vi "Update Relays.vi"(8 "error in (no error)":errorcluster, 10 "MUX Section Ref in":T1 format="%.0x", 11 "Selected MUX Relays":refnum<vi>) -> (0 "error out":errorcluster)   [LabVIEW 2013, in "MUX Custom Device.lvlib"]
uses:
  MUX Custom Device.lvlib
  <vilib>/NI Veristand/Custom Device API/Custom Device Item Ref.ctl
  Relay Channel Data.ctl
  Relay Data.ctl
  Switch.ctl
  MUX Global.vi
  <vilib>/NI Veristand/Custom Device API/Get Item Property (String).vi
  <vilib>/NI Veristand/Custom Device Tools/Custom Device Utility Library/Custom Device Utility Library.lvlib
  <vilib>/NI Veristand/Custom Device API/Custom Device API.lvlib
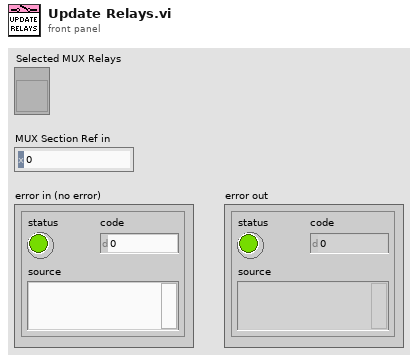
[diagram p1: front panel]
types:
  T1 = typedef "Custom Device API.lvlib/Custom Device Item Ref.ctl" = u64
  T2 = typedef "Relay Status.ctl" = cluster{"Present":bool, "Relay Data":T3}
  T3 = typedef "MUX Custom Device.lvlib/Relay Data.ctl" = cluster{"Relay Name":string, "State":T4}
  T4 = typedef "MUX Custom Device.lvlib/Switch.ctl" = bool
  T5 = typedef "MUX Custom Device.lvlib/Relay Status.ctl" = cluster{"Present":bool, "Relay Data":T3}
  T6 = typedef "MUX Custom Device.lvlib/Relay Channel Data.ctl" = cluster{"Relay Channel Name":string, "Relay Data":T3}
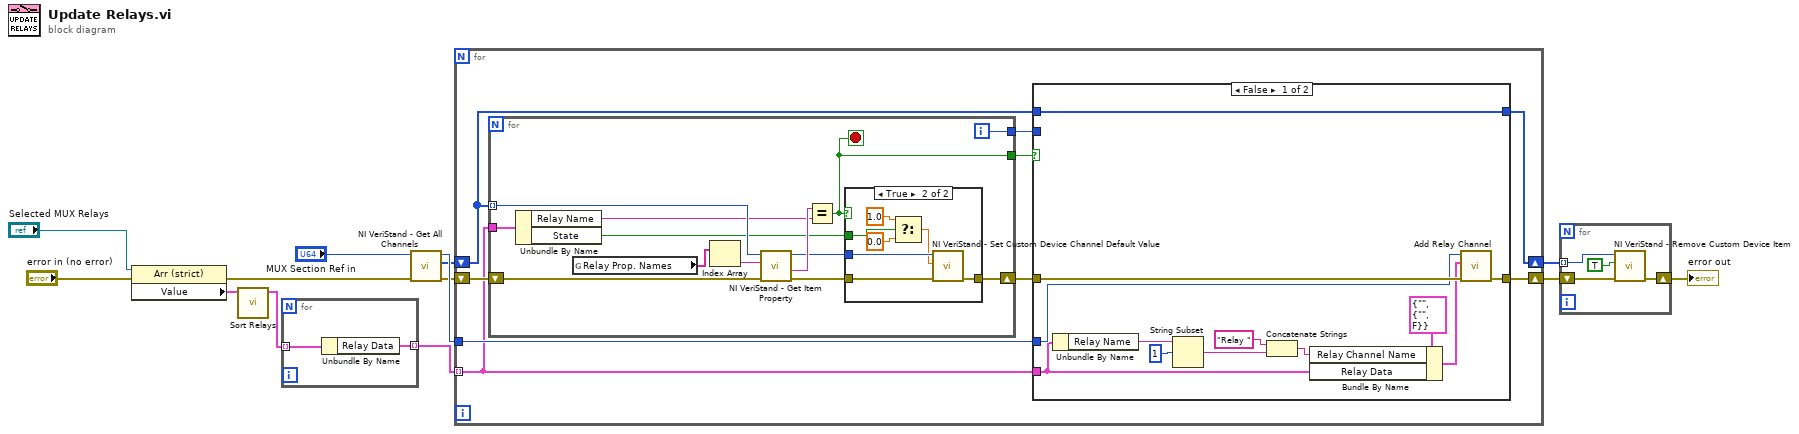
[diagram p0: block diagram]
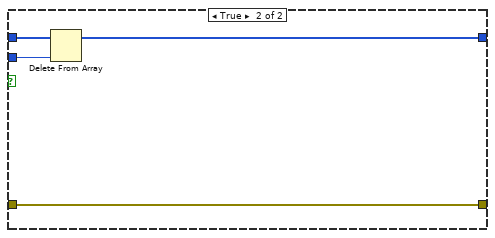
[diagram p2: hidden frame]
diagram:
  n1 = property class="Arr (strict)"(reference="Selected MUX Relays", error in="error in (no error)") -> (error out=w1:errorcluster, "Value"=w12:T2[])  [unwired: 1 out]
  n2 = call "Sort Relays.vi"("Relays"=w12) -> ("Sorted Relays"=w13:T5[])  [unwired: 10 in]
  n3 = for {
    tunnel: w13 -> [w15] mode=indexing
    tunnel: [w14] -> w7 mode=indexing
    n4 = Unbundle By Name(w15) -> ("Relay Data"=w14:T3)
  }
  n5 = call <vilib>:"NI VeriStand - Get All Channels.vi"("error in"=w1, "Section Ref in"="MUX Section Ref in") -> ("error out"=w6:errorcluster, "Channel Refs"=w5:T1[], "Section Ref out"=w8:T1)  [unwired: 6 in, 1 out]
  n6 = for {
    shift-right: [w22] -> w10
    shift-left: w5 -> [w23]
    tunnel: w7 -> [w18] mode=indexing
    tunnel: w8 -> [w20]
    shift-right: [w19] -> w9
    shift-left: w6 -> [w24]
    n7 = for {
      tunnel: w23 -> [w53] mode=indexing
      tunnel: w18 -> [w48]
      shift-right: [w44] -> w21
      shift-left: w24 -> [w49]
      tunnel: [w42] -> w17
      tunnel: [w41] -> w16
      i -> [w42]
      stop <- w41 stop-if-true
      n8 = Unbundle By Name(w48) -> ("Relay Name"=w47:string, "State"=w43:T4)
      n9 = global read "MUX Global.vi" "Relay Prop. Names"() -> (w52:string[])
      n10 = Index Array(array=w52) -> (element=w51:string)  [unwired: 1 in]
      n11 = call-poly <vilib>:"NI VeriStand - Get Item Property.vi"("error in (no error)"=w49, "Property Name"=w51, "Item Ref in"=w53) -> ("error out"=w46:errorcluster, "Value"=w50:string, "Item Ref out"=w45:T1)  [unwired: 5 in, 1 out]
      n12 = Equal?(x=w50, y=w47) -> (x = y?=w41:bool)
      n13 = case shown="True" w41 {
        tunnel: w46 -> [w54 w61]
        tunnel: w45 -> [_ w60]
        tunnel: [w54 w59] -> w44
        tunnel: w43 -> [_ w58]
        frame False {
        }
        frame True {
          n14 = Select(t=1.0, s=w58, f=0.0) -> (s? t:f=w55:dbl)
          n15 = call <vilib>:"NI VeriStand - Set Custom Device Channel Default Value.vi"("error in (no error)"=w61, "Default Value"=w55, "Channel Ref in"=w60) -> ("error out"=w59:errorcluster)  [unwired: 7 in, 1 out]
        }
      }
    }
    n16 = case shown="False" w16 {
      tunnel: w23 -> [w36 w40]
      tunnel: [w36 w39] -> w22
      tunnel: w21 -> [w35 w37]
      tunnel: w20 -> [w34 _]
      tunnel: [w33 w37] -> w19
      tunnel: w18 -> [w30 _]
      tunnel: w17 -> [_ w38]
      frame False {
        n17 = Unbundle By Name(w30) -> ("Relay Name"=w29:string)
        n18 = String Subset(string=w29, offset (0)=1) -> (substring=w27:string)  [unwired: 1 in]
        n19 = Concatenate Strings("Relay " ("string"), w27) -> (w25:string)
        n20 = Bundle By Name(cluster=T6 {"Relay Channel Name"="", "Relay Data"={"Relay Name"="", "State"=FALSE}} ("Relay Channel Data"), "Relay Channel Name"=w25, "Relay Data"=w30) -> (w31:T6)
        n21 = call "Add Relay Channel.vi"("error in (no error)"=w35, "Relay Channel Data"=w31, "MUX Section Ref in"=w34) -> ("error out"=w33:errorcluster)  [unwired: 7 in, 1 out]
      }
      frame True {
        n22 = Delete From Array(array=w40, index=w38) -> (array with subset deleted=w39:T1[])  [unwired: 1 in, 1 out]
      }
    }
  }
  n23 = for {
    tunnel: w10 -> [w65] mode=indexing
    shift-right: [w63] -> w11
    shift-left: w9 -> [w64]
    n24 = call <vilib>:"NI VeriStand - Remove Custom Device Item.vi"("error in (no error)"=w64, "Force Delete (F)"=TRUE, "Item Ref in"=w65) -> ("error out"=w63:errorcluster)  [unwired: 7 in, 1 out]
  }
  "error out" <- w11
